vi "go get xy.vi"() -> ()   [LabVIEW 2016]
uses:
  Classes/Controller/Motion/A3200 Folder/A3200.lvclass
  D:/Gantry_General/Classes/Controller/Motion/Motion Folder/Motion.lvclass
  Classes/Controller/Dispenser/Ultimus V2 Folder/Ultimus V2.lvclass
  Classes/Controller/I-O/NI-DAQ Folder/NI-DAQ.lvclass
  Classes/Controller/Motion/Motion Folder/Motion.lvclass
  Classes/Controller/I-O/I-O Folder/I-O.lvclass
  Classes/Controller/Dispenser/Dispenser Folder/Dispenser.lvclass
panel:
  in  "XYZTheta In":dbl[](array[numeric])=[740.0, 812.0, 61.0, 0.0]
  in  "move to needle position":bool
  out "offset P1-P2":dbl[](array[numeric])=[-219.40879239269793, -67.88363194308386, -7.838721596570402, -1.1025486912928037e-07]
  out "XY center out":dbl[](array[numeric])=[870.025863984025, 828.305856259984]
  out "XY theta out":dbl=-2.841540496462552
  in  "controller in":T1
  in  "go":bool
  in  "stop":bool
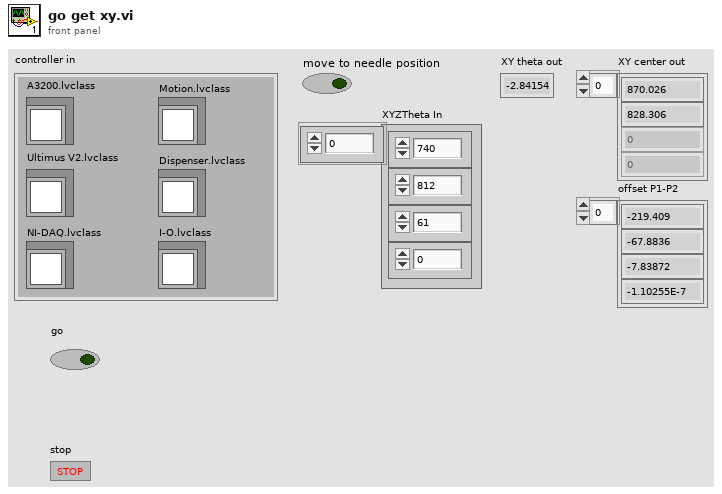
[diagram p1: front panel]
types:
  T1 = cluster{"A3200.lvclass":refnum<class "A3200.lvclass">, "Ultimus V2.lvclass":refnum<class "Ultimus V2.lvclass">, "NI-DAQ.lvclass":refnum<class "NI-DAQ.lvclass">, "Motion.lvclass":refnum<class "Motion.lvclass">, "I-O.lvclass":refnum<class "I-O.lvclass">, "Dispenser.lvclass":refnum<class "Dispenser.lvclass">}
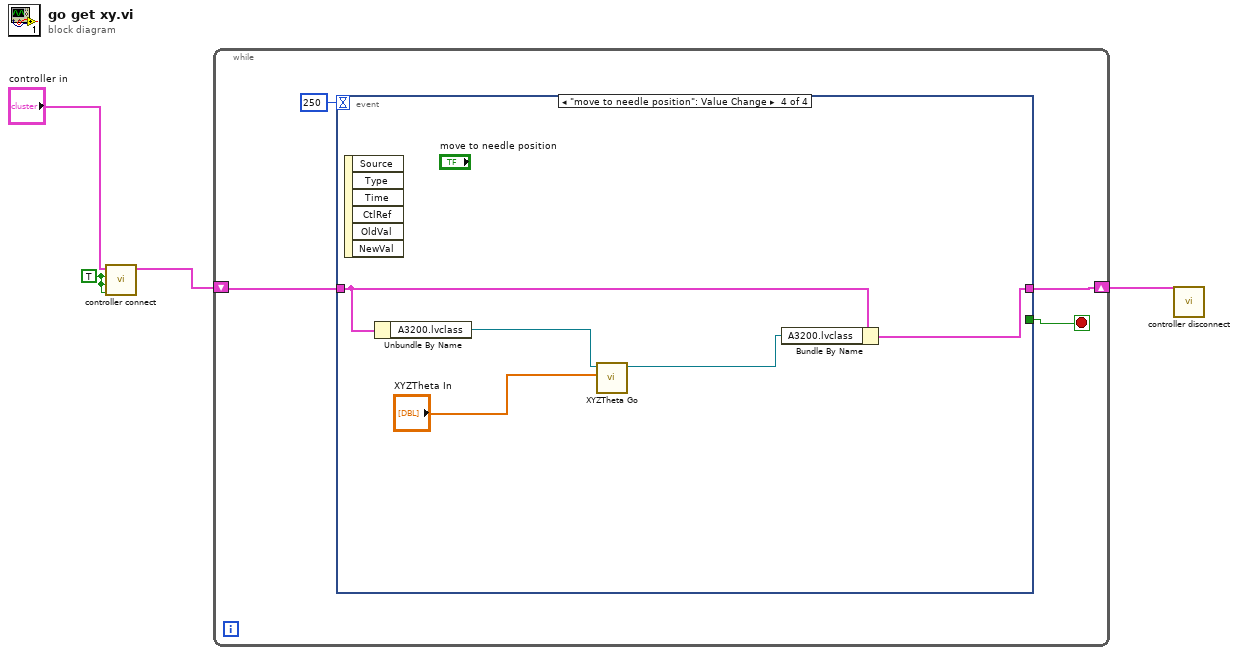
[diagram p0: block diagram]
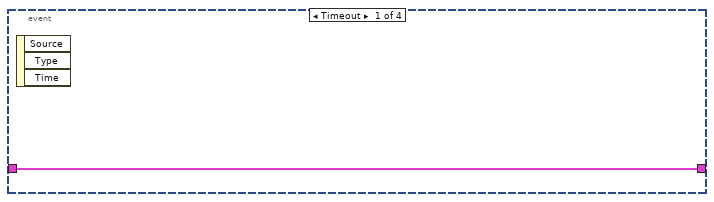
[diagram p2: hidden frame]
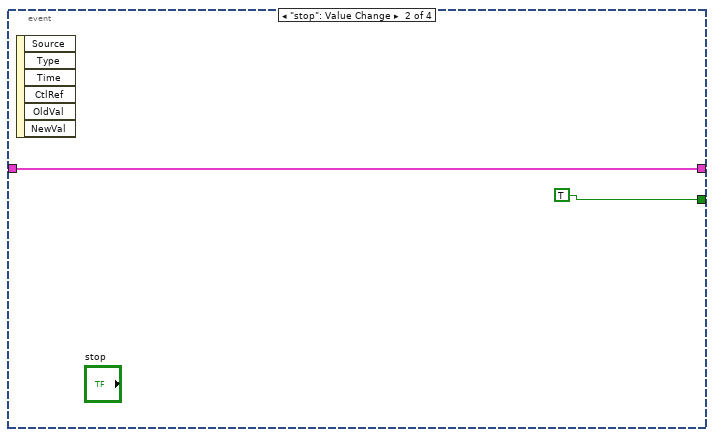
[diagram p3: hidden frame]
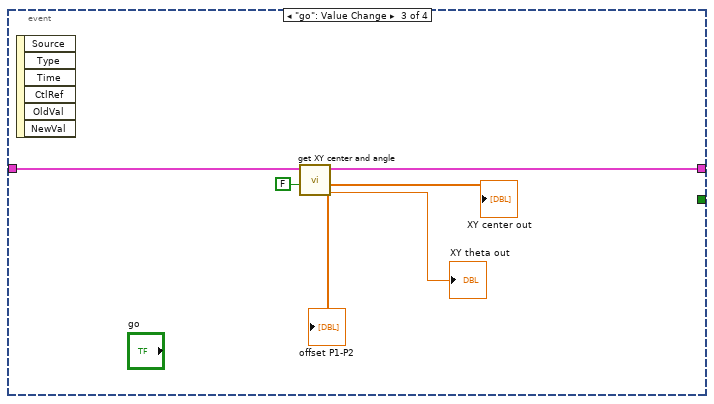
[diagram p4: hidden frame]
diagram:
  w1 = TRUE ("motion on")
  n1 = call "controller connect.vi"("IO on"=w1, "dispencer on"=w1, "motion on"=w1, "controller in"="controller in") -> ("controller out"=w2:T1)  [unwired: 7 in]
  n2 = while {
    shift-right: [w5] -> w4
    shift-left: w2 -> [w6]
    stop <- w7 stop-if-true
    n3 = event shown="[3] \"move to needle position\": Value Change" {
      selector: _ -> [_ _ _ _]
      dyn-events: _ -> [_ _ _ _]
      timeout: 250 -> [_ _ _ _]
      tunnel: [_ TRUE _ _] -> w7
      tunnel: [w9 w10 w17 w20] -> w5
      tunnel: w6 -> [w9 w10 w16 w21]
      event Timeout {
        n4 = event-data() -> ()  [unwired: 1 in, 3 out]
      }
      event "stop": Value Change {
        n5 = event-data() -> ()  [unwired: 1 in, 6 out]
      }
      event "go": Value Change {
        n6 = event-data() -> ()  [unwired: 1 in, 6 out]
        n7 = call "get XY center and angle.vi"("output P1 XY"=FALSE, "controller in"=w16) -> ("XY theta out"=→"XY theta out":dbl, "XY center out"=→"XY center out":dbl[], "controller out"=w17:T1, "offset P1-P2"=→"offset P1-P2":dbl[])  [unwired: 6 in]
      }
      event "move to needle position": Value Change {
        n8 = event-data() -> ()  [unwired: 1 in, 6 out]
        n9 = Unbundle By Name(w21) -> ("A3200.lvclass"=w18:refnum<class "A3200.lvclass">)
        n10 = call "XYZTheta Go.vi"("XYZTheta In"="XYZTheta In", "Motion in"=w18) -> ("Motion out"=w19:refnum<class "A3200.lvclass">)  [unwired: 7 in, 2 out]
        n11 = Bundle By Name(cluster=w21, "A3200.lvclass"=w19) -> (w20:T1)
      }
    }
  }
  n12 = call "controller disconnect.vi"("controller 2"=w4) -> ()  [unwired: 11 in]
